vi "content.vi"(7 "httpRequestID":u32) -> ()   [LabVIEW 2011]
doc: "This VI is a state machine that can be ran from a Browser."
uses:
  server/database/Users/User Record.ctl
  <vilib>/wsapi/NI_WebServices.lvlib
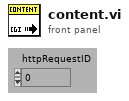
[diagram p1: front panel]
types:
  T1 = typedef "User Record.ctl" = cluster{"ixUser":i32, "sxUsername":string, "sLastName":string, "sFirstName":string, "sEmail":string, "sPassword":string, "tLoginTime":timestamp, "sLoginComputer":string, "fAdministrator":bool, "fRunSequences":bool, "fModifySequences":bool, "fRunScenarios":bool, "fModifyScenarios":bool, "fModifyTemplates":bool, "fModifyUsers":bool, "fModifyStations":bool, "fModifyFields":bool}
  T2 = typedef "Connection Refnum.ctl" = cluster{"Environment Handle":i32, "Connection Handle":i32}
  T3 = typedef "Keyed Array.ctl" = cluster{"keys":string[], "values":string[]}
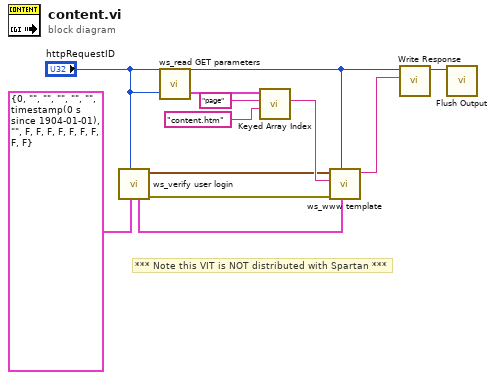
[diagram p0: block diagram]
diagram:
  # "*** Note this VIT is NOT distributed with Spartan ***"
  n1 = call "ws_verify user login.vi"("Required Permisions"=T1 {"ixUser"=0, "sxUsername"="", "sLastName"="", "sFirstName"="", "sEmail"="", "sPassword"="", "tLoginTime"=timestamp(0 s since 1904-01-01), "sLoginComputer"="", "fAdministrator"=FALSE, "fRunSequences"=FALSE, "fModifySequences"=FALSE, "fRunScenarios"=FALSE, "fModifyScenarios"=FALSE, "fModifyTemplates"=FALSE, "fModifyUsers"=FALSE, "fModifyStations"=FALSE, "fModifyFields"=FALSE}, "httpRequestID"="httpRequestID") -> ("error out"=w4:errorcluster, "DB Connection Ref"=w5:T2, "User"=w3:T1)  [unwired: 6 in, 1 out]
  n2 = call "ws_read GET parameters.vi"("httpRequestID"="httpRequestID") -> ("GET query params"=w9:T3)  [unwired: 2 in]
  n3 = call <vilib>:"Keyed Array Index.vi"("default value"="content.htm" ("Template (\"\")"), "key"="page", "array in"=w9) -> ("value"=w8:string)  [unwired: 1 in, 3 out]
  n4 = call "ws_www template.vi"("User"=w3, "httpRequestID"="httpRequestID", "error in (no error)"=w4, "Template (\"\")"=w8, "DB Connection Ref"=w5) -> ("HTTP Template Content"=w6:string)  [unwired: 6 in]
  n5 = call <vilib>:"Write Response.vi"("response string"=w6, "httpRequestID"="httpRequestID") -> ("httpRequestID out"=w7:u32)  [unwired: 8 in, 1 out]
  n6 = call <vilib>:"Flush Output.vi"("httpRequestID"=w7) -> ()  [unwired: 9 in, 2 out]
